vi "GLIMPSE Initialize.vi"() -> ()   [LabVIEW 2011]
doc: "This VI sets up certain global variables for the rest of GLIMPSE. It is designed to be called only once per execution."
uses:
  GLIMPSE Globals.vi
  Instance           6 26Saved   GLIMPSE Initialize .vi
panel:
  out "Disk Drive":path
  out "Acquisition drive\nfree space (Gb)":dbl format="%.2f"
  out "Labview Hardware Configuration File":path
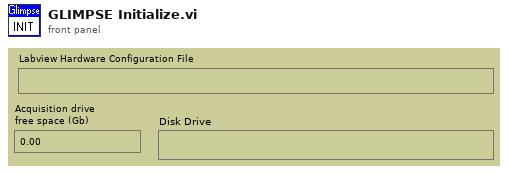
[diagram p1: front panel]
types:
  T1 = enum32{"8 bits", "16 bits", "Float", "Complex", "RGB Chunky", "Compressed"}
  T2 = typedef "IMAQ Image.ctl" = refnum<image>
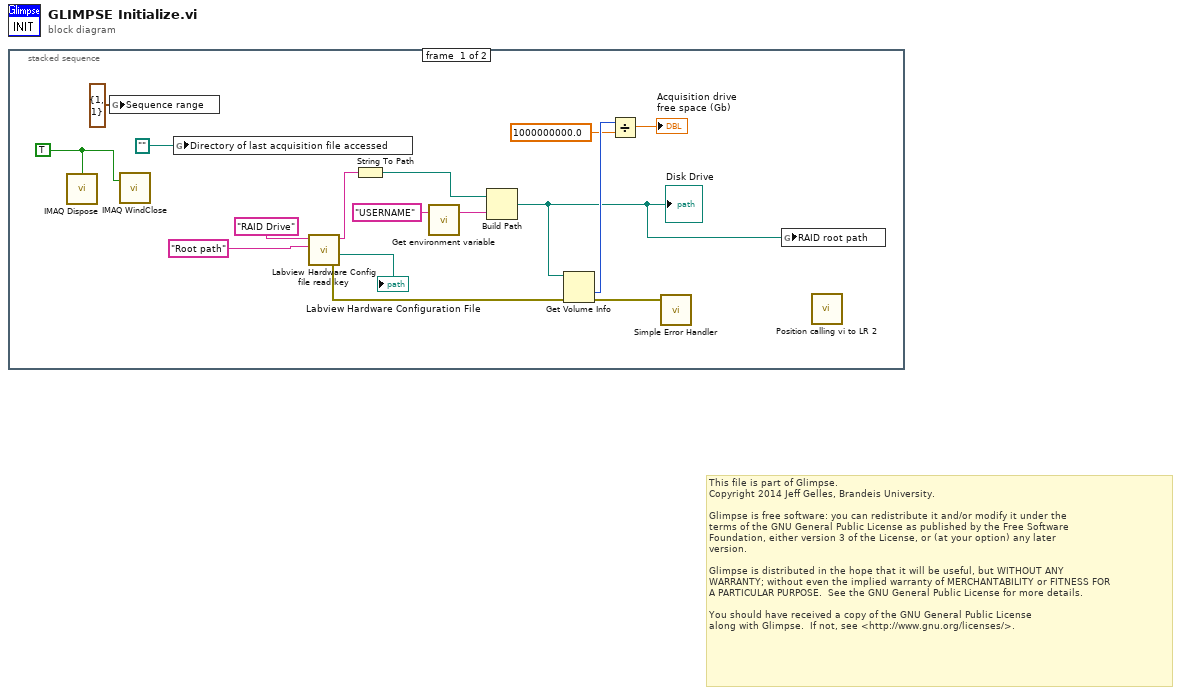
[diagram p0: block diagram]
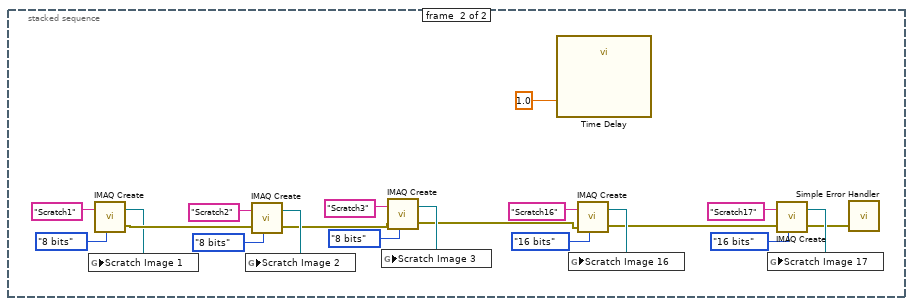
[diagram p2: hidden frame]
diagram:
  # "This file is part of Glimpse. \nCopyright 2014 Jeff Gelles, Brandeis University.    \n\nGlimpse is free software: you can redistribute it and/or modify it under the \nterms of the GNU General Public License as published by the Free Software \nFoundation, either version 3 of the License, or (at your option) any later \nversion.\n\nGlimpse is distributed in the hope that it will be useful, but WITHOUT ANY \nWARRANTY; without even the implied warranty of MERCHANTABILITY or FITNESS FOR \nA PARTICULAR PURPOSE.  See the GNU General Public License for more details.\n\nYou should have received a copy of the GNU General Public License\nalong with Glimpse.  If not, see <http://www.gnu.org/licenses/>."
  n1 = stacked-sequence {
    frame #0 {
      w5 = TRUE ("All Images? (No)")
      n2 = call "IMAQ Dispose"("All Images? (No)"=w5) -> ()  [unwired: 2 in, 4 out]
      n3 = global write "GLIMPSE Globals.vi" "Sequence range"(cluster{i16, i16} {1, 1} ("Sequence range")) -> ()
      n4 = call "IMAQ WindClose"("Close All Windows (False)"=w5) -> ()  [unwired: 2 in, 4 out]
      n5 = global write "GLIMPSE Globals.vi" "Directory of last acquisition file accessed"(path "") -> ()
      n6 = call "Labview Hardware Config file read key.vi"("key name in"="Root path", "section"="RAID Drive") -> ("error out"=w11:errorcluster, "File read"=→"Labview Hardware Configuration File":path, "key vlue out"=w13:string)  [unwired: 2 in, 2 out]
      n7 = String To Path(string=w13) -> (path=w2:path)
      n8 = call "Get environment variable.vi"("Variable name"="USERNAME") -> ("Value"=w3:string)  [unwired: 2 out]
      n9 = Build Path(base path=w2, name or relative path=w3) -> (appended path=w1:path)
      "Disk Drive" <- w1
      n10 = Get Volume Info(8:w11, 11:w1) -> (0:w6:errorcluster, 1:w9:i64)  [unwired: 4 out]
      n11 = Divide(x=w9, y=1000000000.0) -> (x/y=→"Acquisition drive\nfree space (Gb)":dbl)
      n12 = call <vilib>:"Simple Error Handler.vi"("error in (no error)"=w6) -> ()  [unwired: 1 in, 8 out]
      n13 = global write "GLIMPSE Globals.vi" "RAID root path"(w1) -> ()
      n14 = call "Position calling vi to LR 2.vi"() -> ()  [unwired: 2 in, 4 out]
    }
    frame #1 {
      n15 = call "IMAQ Create"("Image Name"="Scratch1", "Image Type"=T1."8 bits") -> ("New Image"=w32:T2, "error out"=w35:errorcluster)  [unwired: 2 in, 1 out]
      n16 = global write "GLIMPSE Globals.vi" "Scratch Image 1"(w32) -> ()
      n17 = call "IMAQ Create"("Image Name"="Scratch2", "Image Type"=T1."8 bits", "error in (no error)"=w35) -> ("New Image"=w31:T2, "error out"=w24:errorcluster)  [unwired: 1 in, 1 out]
      n18 = global write "GLIMPSE Globals.vi" "Scratch Image 2"(w31) -> ()
      n19 = call "IMAQ Create"("Image Name"="Scratch3", "Image Type"=T1."8 bits", "error in (no error)"=w24) -> ("New Image"=w27:T2, "error out"=w23:errorcluster)  [unwired: 1 in, 1 out]
      n20 = global write "GLIMPSE Globals.vi" "Scratch Image 3"(w27) -> ()
      n21 = call "Time Delay"("Delay Time (s)"=1.0) -> ()  [unwired: 1 in, 10 out]
      n22 = call "IMAQ Create"("Image Name"="Scratch16", "Image Type"=T1."16 bits", "error in (no error)"=w23) -> ("New Image"=w30:T2, "error out"=w18:errorcluster)  [unwired: 1 in, 1 out]
      n23 = global write "GLIMPSE Globals.vi" "Scratch Image 16"(w30) -> ()
      n24 = call "IMAQ Create"("Image Name"="Scratch17", "Image Type"=T1."16 bits", "error in (no error)"=w18) -> ("New Image"=w20:T2, "error out"=w19:errorcluster)  [unwired: 1 in, 1 out]
      n25 = global write "GLIMPSE Globals.vi" "Scratch Image 17"(w20) -> ()
      n26 = call <vilib>:"Simple Error Handler.vi"("error in (no error)"=w19) -> ()  [unwired: 1 in, 8 out]
    }
  }
